vi "Teste de conexão.vi"() -> ()   [LabVIEW 2016]
uses:
  <vilib>/addons/_JKI Toolkits/Caraya/classes/Test/Test.lvclass
  <vilib>/addons/_JKI Toolkits/Caraya/classes/Assert/Assert.lvclass
panel:
  out "error out":errorcluster
  in  "error in (no error)":errorcluster
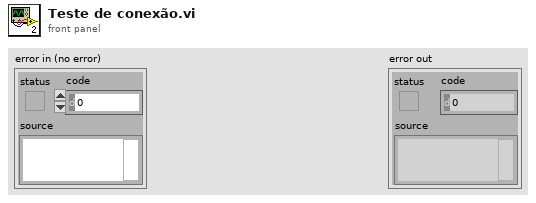
[diagram p1: front panel]
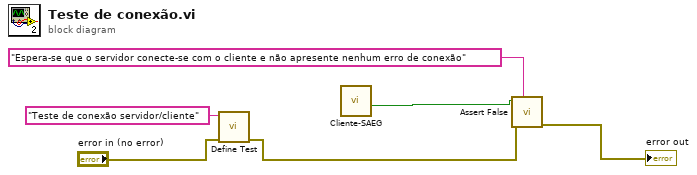
[diagram p0: block diagram]
diagram:
  n1 = call <vilib>:"Define Test.vi"("error in (no error)"="error in (no error)", "Label (VI Title)"="Teste de conexão servidor/cliente") -> ("error out"=w4:errorcluster)  [unwired: 9 in]
  n2 = call "Cliente-SAEG.vi"() -> ("status"=w1:bool)  [unwired: 11 in]
  n3 = call <vilib>:"Assert False.vi"("Label"="Espera-se que o servidor conecte-se com o cliente e não apresente nenhum erro de conexão", "error in (no error)"=w4, "False?"=w1) -> ("error out"=→"error out":errorcluster)  [unwired: 8 in]
